vi "Initialize Interaction Map.vi"(9 "interaction name":string, 10 "incoming interactions":map{string, map{string, i32}}(c390), 11 "interaction map in":T1) -> (3 "interaction map out":T1)   [LabVIEW 2019, in "HLA Custom Device Engine.lvlib"]
uses:
  HLA Custom Device Engine.lvlib
  map_interaction_value.ctl
  map_attr_param_data.ctl
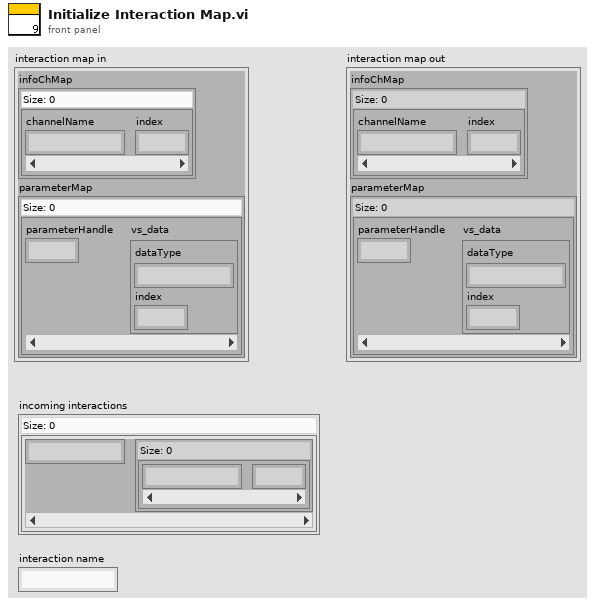
[diagram p1: front panel]
types:
  T1 = typedef "HLA Custom Device Engine.lvlib/map_interaction_value.ctl" = cluster{"infoChMap":map{string, i32}, "parameterMap":map{u64, T2}}
  T2 = typedef "HLA Custom Device Engine.lvlib/map_attr_param_data.ctl" = cluster{"dataType":string, "index":i32}
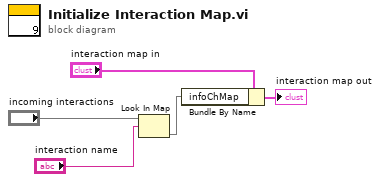
[diagram p0: block diagram]
diagram:
  n1 = Look In Map(map="incoming interactions", key="interaction name") -> (value=w3:map{string, i32})  [unwired: 1 in, 1 out]
  n2 = Bundle By Name(cluster="interaction map in", "infoChMap"=w3) -> (→"interaction map out":T1)
